vi "COMMAND ROM FILE.vi"() -> ()   [LabVIEW 2020]
uses:
  <instrlib>/Agilent B2900 Series/Agilent B2900 Series.lvlib
panel:
  in  "write buffer":string
  out "Measurement":dbl
  out "error out":errorcluster
  out "read buffer":string
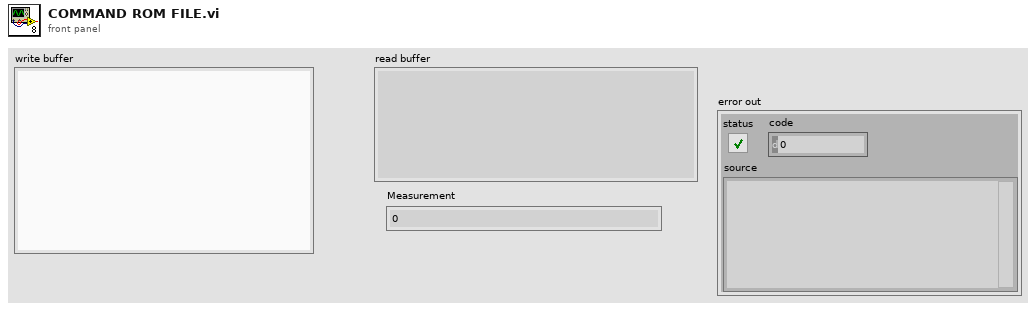
[diagram p1: front panel]
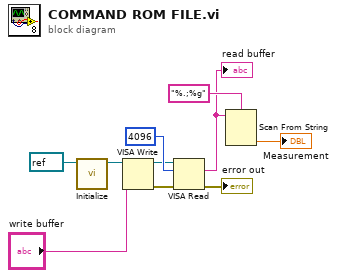
[diagram p0: block diagram]
diagram:
  n1 = call <instrlib>:"Initialize.vi"("VISA resource name"=refnum<visa-resource-name> "USB0::0x0957::0x8E18::MY51140695::INSTR") -> ("VISA resource name out"=w5:refnum<visa-resource-name>)  [unwired: 9 in, 1 out]
  n2 = VISA Write(VISA resource name=w5, write buffer="write buffer") -> (VISA resource name out=w9:refnum<visa-resource-name>, error out=w8:errorcluster)  [unwired: 1 in, 1 out]
  n3 = VISA Read(VISA resource name=w9, byte count=u32 4096, error in (no error)=w8) -> (read buffer=w2:string, error out=→"error out":errorcluster)  [unwired: 2 out]
  "read buffer" <- w2
  n4 = Scan From String(format string="%.;%g", input string=w2) -> (output 1=→"Measurement":dbl)  [unwired: 3 in, 3 out]
